vi "Write Calibration info.vi"(10 "Calibration info":string, 11 "Vector Network Analyzer in":refnum<class "Vector Network Analyzer.lvclass">) -> (3 "Vector Network Analyzer out":refnum<class "Vector Network Analyzer.lvclass">)   [LabVIEW 2020, in "Vector Network Analyzer.lvclass"]
uses:
  Vector Network Analyzer.lvclass
  Vector Network Analyzer.lvclass/Vector Network Analyzer.ctl
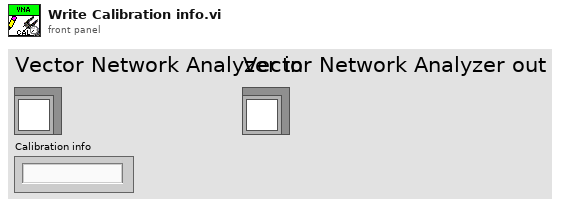
[diagram p1: front panel]
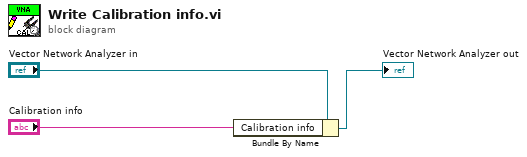
[diagram p0: block diagram]
diagram:
  n1 = Bundle By Name(cluster="Vector Network Analyzer in", "Calibration info"="Calibration info") -> (→"Vector Network Analyzer out":refnum<class "Vector Network Analyzer.lvclass">)
